vi "get and set immutable.vi"() -> ()   [LabVIEW 2013]
uses:
  errors/severity.ctl
  errors/const messagename.vi
  errors/const exceptioncausename.vi
  errors/const sourcename.vi
  errors/exception.lvlib
panel:
  out "message":string
  out "call chain ok":bool
  out "src2 ok":bool
  out "msg2 ok":bool
  out "msg1 ok":bool
  out "src1 ok":bool
  out "cause ok":bool
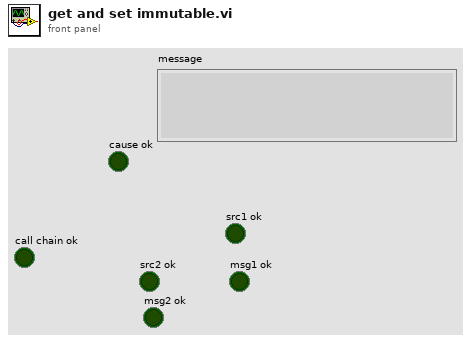
[diagram p1: front panel]
types:
  T1 = typedef "exception.lvlib/severity.ctl" = enum8{"unspecified", "operation failed", "data corruption", "system corruption", "critical unknown state"}
  T2 = typedef "exception.lvlib/exception.ctl" = cluster{"code":i32, "context":T3, "properties":variant}
  T3 = typedef "exception.lvlib/context.ctl" = enum16{"developer", "user interface", "standard", "limited", "deterministic"}
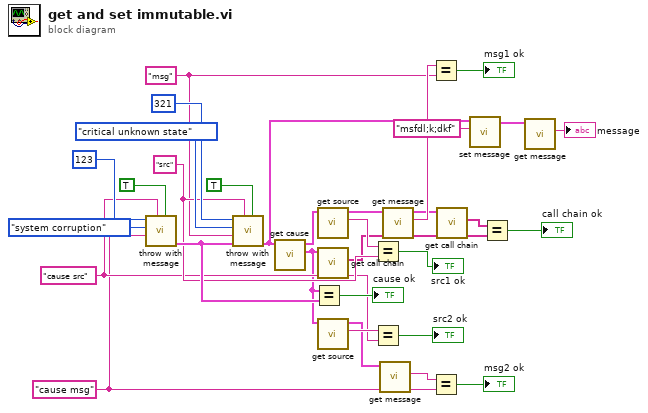
[diagram p0: block diagram]
diagram:
  w6 = "cause msg" ("message")
  w12 = "cause src" ("source")
  w5 = "msg" ("message")
  w20 = "src" ("source")
  n1 = call "throw with message.vi"("call chain?"=TRUE, "source"=w12, "message"=w6, "severity"=severity."system corruption", "code"=123) -> ("exception out"=w26:T2)  [unwired: 6 in]
  n2 = call "throw with message.vi"("call chain?"=TRUE, "source"=w20, "exception in"=w26, "message"=w5, "severity"=severity."critical unknown state", "code"=321) -> ("exception out"=w4:T2)  [unwired: 5 in]
  n3 = call "get cause.vi"("exception in"=w4) -> ("cause"=w10:T2, "exception out"=w24:T2)  [unwired: 9 in]
  n4 = Equal?(x=w10, y=w26) -> (x = y?=→"cause ok":bool)
  n5 = call "get source.vi"("exception in"=w24) -> ("source"=w21:string, "exception out"=w19:T2)  [unwired: 9 in]
  n6 = call "get call chain.vi"("exception in"=w10) -> ("call chain"=w8:string[])  [unwired: 9 in, 1 out]
  n7 = call "get source.vi"("exception in"=w10) -> ("source"=w16:string, "exception out"=w13:T2)  [unwired: 9 in]
  n8 = Equal?(x=w21, y=w20) -> (x = y?=→"src1 ok":bool)
  n9 = Equal?(x=w16, y=w12) -> (x = y?=→"src2 ok":bool)
  n10 = call "get message.vi"("exception in"=w13) -> ("message"=w17:string)  [unwired: 9 in, 1 out]
  n11 = call "get message.vi"("exception in"=w19) -> ("message"=w18:string, "exception out"=w11:T2)  [unwired: 9 in]
  n12 = Equal?(x=w18, y=w5) -> (x = y?=→"msg1 ok":bool)
  n13 = Equal?(x=w17, y=w6) -> (x = y?=→"msg2 ok":bool)
  n14 = call "get call chain.vi"("exception in"=w11) -> ("call chain"=w7:string[])  [unwired: 9 in, 1 out]
  n15 = call "set message.vi"("message"="msfdl;k;dkf", "exception in"=w4) -> ("exception out"=w2:T2)  [unwired: 9 in]
  n16 = Equal?(x=w7, y=w8) -> (x = y?=→"call chain ok":bool)
  n17 = call "get message.vi"("exception in"=w2) -> ("message"=→"message":string)  [unwired: 9 in, 1 out]
